vi "FG LocalPose.vi"(1 "FG Action (Read)":T3, 2 "LocalPose in":T1) -> (0 "LocalPose out":T1)   [LabVIEW 2009]
uses:
  cRIO/Functional Global Variables/Actions for FG's.ctl
  LocalPose.ctl
  TimeRec.ctl
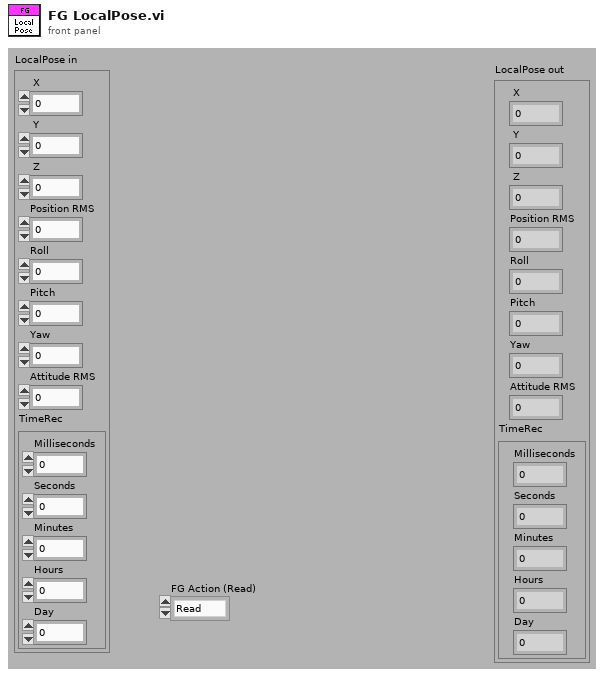
[diagram p1: front panel]
types:
  T1 = typedef "LocalPose.ctl" = cluster{" X":dbl, " Y":dbl, " Z":dbl, "Position RMS":dbl, "Roll":dbl, "Pitch":dbl, "Yaw":dbl, "Attitude RMS":dbl, "TimeRec":T2}
  T2 = typedef "TimeRec.ctl" = cluster{"Milliseconds":u32, "Seconds":u32, "Minutes":u32, "Hours":u32, "Day":u32}
  T3 = typedef "Actions for FG's.ctl" = enum16{"Read", "Write"}
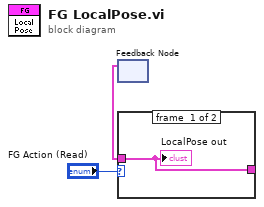
[diagram p0: block diagram]
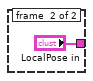
[diagram p2: hidden frame]
diagram:
  n1 = feedback #1() -> (w1:T1)  [unwired: 1 in]
  n2 = case shown="\"Read\", Default" "FG Action (Read)" {
    tunnel: w1 -> [w4 _]
    tunnel: [w4 "LocalPose in"] -> w2
    frame #0 {
      "LocalPose out" <- w4
    }
    frame #1 {
    }
  }
